vi "Open SenseHat.Joystick.vi"(8 "error in (no error)":errorcluster, 11 "LINX Resource":T1) -> (0 "error out":errorcluster, 3 "senseHatJoystick out":refnum<class "RPI.SenseHat.Joystick.lvclass">)   [LabVIEW 2020, in "RPI.SenseHat.Joystick.lvlib" / "RPI.SenseHat.Joystick.lvclass"]
uses:
  RPI.SenseHat.Joystick.lvclass
  <vilib>/MakerHub/LINX/Private/Type Defs/LINX Ref.ctl
  <vilib>/MakerHub/LINX/Private/Type Defs/Platform.ctl
  <vilib>/MakerHub/LINX/Private/Type Defs/Interface.ctl
  <vilib>/MakerHub/LINX/Private/Device/Type Defs/LINX Device Config.ctl
  <vilib>/MakerHub/LINX/Private/Device/Type Defs/TCP Config.ctl
  <vilib>/MakerHub/LINX/Private/Device/Type Defs/Channels.ctl
  TypeDefs/Key State.ctl
  RPI.SenseHat.Joystick.lvclass/RPI.SenseHat.Joystick.ctl
  RPI/Classes/mainI2CDevice/mainI2CDevice.lvclass
  RPI.SenseHat.Joystick.lvlib
  <vilib>/MakerHub/LINX/LMH-LINX.lvlib
  <vilib>/MakerHub/LINX/Private/Device/Device.lvlib
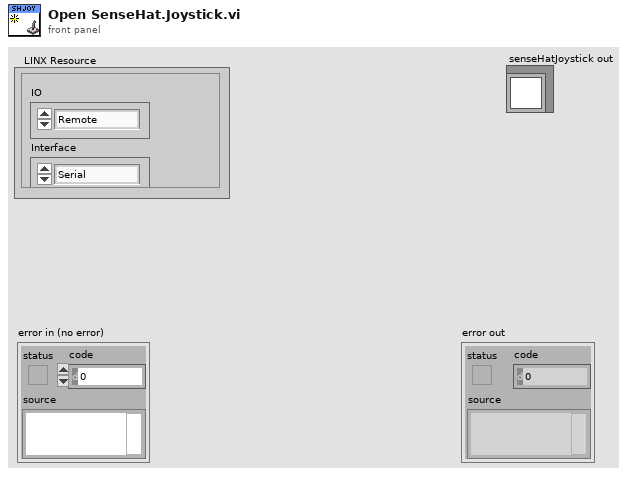
[diagram p1: front panel]
types:
  T1 = typedef "LMH-LINX.lvlib/LINX Ref.ctl" = cluster{"IO":T2, "Interface":T3, "LINX Device Config":T4}
  T2 = typedef "LMH-LINX.lvlib/Platform.ctl" = enum16{"Remote", "Local"}
  T3 = typedef "LMH-LINX.lvlib/Interface.ctl" = enum16{"Serial", "TCP"}
  T4 = typedef "LMH-LINX.lvlib/Device.lvlib/LINX Device Config.ctl" = cluster{"Interface":T3, "COM Port":refnum<visa-resource-name>, "TCP Configuration":T5, "Device Family":u8, "Device ID":u8, "Device Name":string, "TCP Ref":refnum<k5>, "Channels":T6}
  T5 = typedef "LMH-LINX.lvlib/Device.lvlib/TCP Config.ctl" = cluster{"IP Address":string, "Port":u16}
  T6 = typedef "LMH-LINX.lvlib/Channels.ctl" = cluster{"DI":u8[], "DO":u8[], "AI":u8[], "AO":u8[], "PWM":u8[], "QE":u8[], "UART":u8[], "I2C 2":u8[], "SPI":u8[], "CAN":u8[], "Servo":u8[], "AI Ref (V)":dbl, "AI Resolution (Bits)":u8, "AO Ref (V)":dbl, "AO Resolution (Bits)":u8}
  T7 = typedef "RPI.SenseHat.Joystick.lvlib/Key State.ctl" = enum16{"Released", "Pressing", "Pressed", "Releasing"}
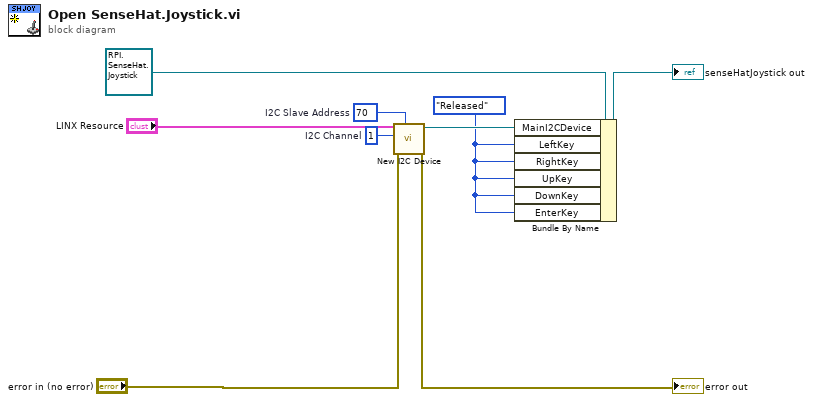
[diagram p0: block diagram]
diagram:
  w1 = Key_State."Released" ("DownKey")
  w2 = u8 70  # I2C Slave Address
  w3 = u8 1  # I2C Channel
  n1 = call "New I2C Device.vi"("I2C Slave Address"=w2, "error in (no error)"="error in (no error)", "I2C Channel"=w3, "object in"="LINX Resource") -> ("error out"=→"error out":errorcluster, "mainI2CDevice out"=w4:refnum<class "mainI2CDevice.lvclass">)  [unwired: 6 in]
  n2 = Bundle By Name(cluster=refnum<class "RPI.SenseHat.Joystick.lvclass"> refnum ("senseHatJoystick in"), "MainI2CDevice"=w4, "LeftKey"=w1, "RightKey"=w1, "UpKey"=w1, "DownKey"=w1, "EnterKey"=w1) -> (→"senseHatJoystick out":refnum<class "RPI.SenseHat.Joystick.lvclass">)
